vi "Create.vi"(8 "error in":errorcluster, 11 "Msg in":refnum<class "Msg.lvclass">) -> (0 "error out":errorcluster, 3 "Msg out":refnum<class "Msg.lvclass">)   [LabVIEW 2020, in "_Rescript.lvlib" / "Msg.lvlib" / "Msg.lvclass"]
uses:
  Msg.lvclass
  Msg.lvclass/Msg.ctl
  _Shared/Project Stuff/Project Stuff.lvclass/Project Stuff.ctl
  _Shared/Name Specs/Name Specs.lvclass/Name Specs.ctl
  _Shared/Name Specs/Name Specs.lvclass
  _Shared/Project Stuff/Project Stuff.lvclass
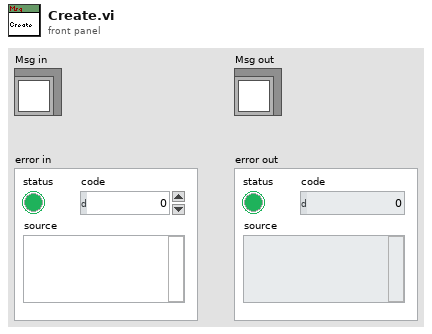
[diagram p1: front panel]
types:
  T1 = typedef "_Shared.lvlib/Name Stuff.ctl" = cluster{"Type (Enum)":T2, "Type (String)":string, "Name Library File Path":path, "Name":string, "Name Type":string}
  T2 = typedef "_Shared.lvlib/Type.ctl" = enum16{"Actor", "Msg"}
  T3 = typedef "_Rescript.lvlib/Msg.lvlib/Msg.lvclass/Name.ctl" = cluster{"Name VI (Lib)":refnum<vi>, "Init Msg VI (Lib)":refnum<vi>, "Call VI (Lib)":refnum<vi>, "Recurse VI (Lib)":refnum<vi>, "Tell Self VI (Lib)":refnum<vi>, "Tell Parent VI (Lib)":refnum<vi>, "Tell Child VI (Lib)":refnum<vi>, "Tell Reply VI (Lib)":refnum<vi>}
  T4 = typedef "_Rescript.lvlib/Msg.lvlib/Msg.lvclass/Name Msg.ctl" = cluster{"Execute VI (Class)":refnum<vi>}
  T5 = typedef "_Rescript.lvlib/Msg.lvlib/Msg.lvclass/Name jettl Msg.ctl" = cluster{"Name VI (Interface)":refnum<vi>}
  T6 = typedef "_Rescript.lvlib/Msg.lvlib/Msg.lvclass/Name Msg IO.ctl" = cluster{"PD Control (Class)":refnum<vi>, "PD Cluster (Class)":refnum<vi>, "Init Msg IO VI (Class)":refnum<vi>, "Read Msg IO VI (Class)":refnum<vi>, "Init Msg IO VI (Lib)":refnum<vi>, "Read Msg IO VI (Lib)":refnum<vi>, "Terminal Attributes (Init)":T7, "Terminal Attributes (Read)":T7}
  T7 = typedef "_Rescript.lvlib/Terminal Attributes.ctl" = map{i32, T8}
  T8 = typedef "_Rescript.lvlib/Attributes.ctl" = cluster{"Control":refnum<vi>, "Wire Rule":enum16{"Invalid Wire Rule", "Required", "Recommended", "Optional", "Dynamic Dispatch"}}
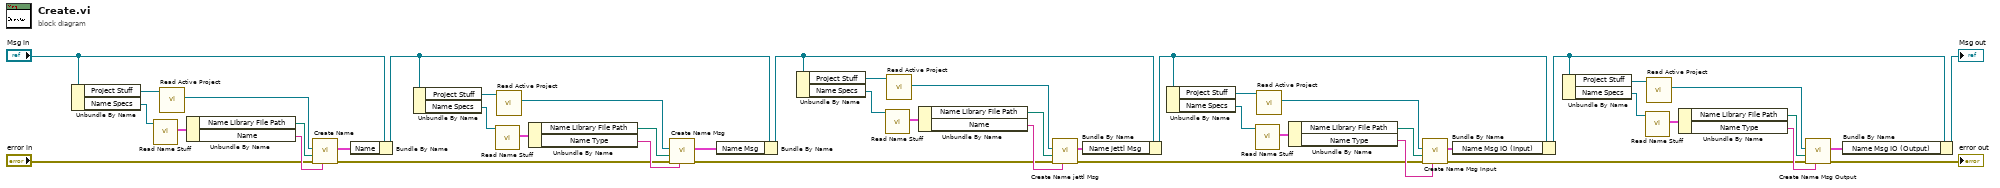
[diagram p0: block diagram]
diagram:
  n1 = Unbundle By Name("Msg in") -> ("Project Stuff"=w23:refnum<class "Project Stuff.lvclass">, "Name Specs"=w30:refnum<class "Name Specs.lvclass">)
  n2 = call "Read Name Stuff.vi"("Name Specs in"=w30) -> ("Name Stuff"=w29:T1)  [unwired: 10 in]
  n3 = call "Read Active Project.vi"("Project Stuff in"=w23) -> ("Active Project"=w20:refnum<vi>)  [unwired: 10 in]
  n4 = Unbundle By Name(w29) -> ("Name Library File Path"=w21:path, "Name"=w22:string)
  n5 = call "Create Name.vi"("Name"=w22, "error in"="error in", "Name Library File Path"=w21, "Active Project"=w20) -> ("error out"=w18:errorcluster, "Name"=w28:T3)  [unwired: 6 in]
  n6 = Bundle By Name(cluster="Msg in", "Name"=w28) -> (w5:refnum<class "Msg.lvclass">)
  n7 = Unbundle By Name(w5) -> ("Project Stuff"=w42:refnum<class "Project Stuff.lvclass">, "Name Specs"=w43:refnum<class "Name Specs.lvclass">)
  n8 = call "Read Name Stuff.vi"("Name Specs in"=w43) -> ("Name Stuff"=w44:T1)  [unwired: 10 in]
  n9 = call "Read Active Project.vi"("Project Stuff in"=w42) -> ("Active Project"=w41:refnum<vi>)  [unwired: 10 in]
  n10 = Unbundle By Name(w44) -> ("Name Library File Path"=w40:path, "Name Type"=w39:string)
  n11 = call "Create Name Msg.vi"("Name Msg"=w39, "error in"=w18, "Name Library File Path"=w40, "Active Project"=w41) -> ("error out"=w17:errorcluster, "Name Msg"=w38:T4)  [unwired: 6 in]
  n12 = Bundle By Name(cluster=w5, "Name Msg"=w38) -> (w4:refnum<class "Msg.lvclass">)
  n13 = Unbundle By Name(w4) -> ("Project Stuff"=w25:refnum<class "Project Stuff.lvclass">, "Name Specs"=w47:refnum<class "Name Specs.lvclass">)
  n14 = call "Read Name Stuff.vi"("Name Specs in"=w47) -> ("Name Stuff"=w46:T1)  [unwired: 10 in]
  n15 = call "Read Active Project.vi"("Project Stuff in"=w25) -> ("Active Project"=w24:refnum<vi>)  [unwired: 10 in]
  n16 = Unbundle By Name(w46) -> ("Name Library File Path"=w27:path, "Name"=w26:string)
  n17 = call "Create Name jettl Msg.vi"("Name"=w26, "error in"=w17, "Name Library File Path"=w27, "Active Project"=w24) -> ("error out"=w8:errorcluster, "Name jettl Msg"=w45:T5)  [unwired: 6 in]
  n18 = Bundle By Name(cluster=w4, "Name jettl Msg"=w45) -> (w3:refnum<class "Msg.lvclass">)
  n19 = Unbundle By Name(w3) -> ("Project Stuff"=w15:refnum<class "Project Stuff.lvclass">, "Name Specs"=w13:refnum<class "Name Specs.lvclass">)
  n20 = call "Read Name Stuff.vi"("Name Specs in"=w13) -> ("Name Stuff"=w14:T1)  [unwired: 10 in]
  n21 = call "Read Active Project.vi"("Project Stuff in"=w15) -> ("Active Project"=w12:refnum<vi>)  [unwired: 10 in]
  n22 = Unbundle By Name(w14) -> ("Name Library File Path"=w11:path, "Name Type"=w10:string)
  n23 = call "Create Name Msg Input.vi"("Name Msg"=w10, "error in"=w8, "Name Library File Path"=w11, "Active Project"=w12) -> ("error out"=w7:errorcluster, "Name Msg IO (Input)"=w9:T6)  [unwired: 6 in]
  n24 = Bundle By Name(cluster=w3, "Name Msg IO (Input)"=w9) -> (w2:refnum<class "Msg.lvclass">)
  n25 = Unbundle By Name(w2) -> ("Project Stuff"=w37:refnum<class "Project Stuff.lvclass">, "Name Specs"=w36:refnum<class "Name Specs.lvclass">)
  n26 = call "Read Name Stuff.vi"("Name Specs in"=w36) -> ("Name Stuff"=w35:T1)  [unwired: 10 in]
  n27 = call "Read Active Project.vi"("Project Stuff in"=w37) -> ("Active Project"=w34:refnum<vi>)  [unwired: 10 in]
  n28 = Unbundle By Name(w35) -> ("Name Library File Path"=w33:path, "Name Type"=w32:string)
  n29 = call "Create Name Msg Output.vi"("Name Msg"=w32, "error in"=w7, "Name Library File Path"=w33, "Active Project"=w34) -> ("error out"=→"error out":errorcluster, "Name Msg IO (Output)"=w31:T6)  [unwired: 6 in]
  n30 = Bundle By Name(cluster=w2, "Name Msg IO (Output)"=w31) -> (→"Msg out":refnum<class "Msg.lvclass">)
